vi "OP600ZP_BOITE_DIALOGUE.vi"(0 "Enable":bool=TRUE caption="Activer", 5 "error in (no error)":errorcluster caption="entrée d'erreur (pas d'erreur)") -> (11 "Factory Temperature":dbl format="%#g", 12 "Min Cell Temperature":dbl format="%#g", 13 "Max Cell Temperature":dbl format="%#g", 14 "Min Cell Voltage":dbl format="%#g", 15 "Max Cell Voltage":dbl format="%#g", 16 "Battery Voltage":dbl format="%#g", 17 "PARK Mode OK?":bool, 18 "OK":bool, 19 "error out":errorcluster caption="sortie d'erreur")   [LabVIEW 2020]
doc: "Affiche une boîte de dialogue standard qui invite l'utilisateur à entrer des informations, telles qu'un nom d'utilisateur et un mot de passe.\n--------------------\n\nCe VI Express est configuré comme suit :\n\nMessage à afficher à l'utilisateur :Saisir les valeur suivantes :\nLes entrées sont : \nCase à cocher : PARK Mode OK?\nNombre : Battery Voltage\nNombre : Max Cell Voltage\nNombre : Min Cell Voltage\nNombre : Max Cell Temperature\nNombre : Min Cell Temperature\nNombre : Factory Temperature"
panel:
  out "SOH":dbl caption="Factory Temperature" format="%#g"
  out "SOC":dbl caption="Factory Temperature" format="%#g"
  in  "SOH":dbl caption="Factory Temperature" format="%#g"
  in  "SOC":dbl caption="Factory Temperature" format="%#g"
  in  "Factory Temperature":dbl format="%#g"
  in  "Min Cell Temperature":dbl format="%#g"
  in  "Max Cell Temperature":dbl format="%#g"
  in  "Min Cell Voltage":dbl format="%#g"
  in  "Max Cell Voltage":dbl format="%#g"
  in  "Battery Voltage":dbl format="%#g"
  in  "PARK Mode OK?":bool
  out "String":string="Saisir les valeur suivantes :" caption="Chaîne"
  in  "Cancel":bool caption="Annuler"
  in  "OK2":bool
  in  "OK1":bool
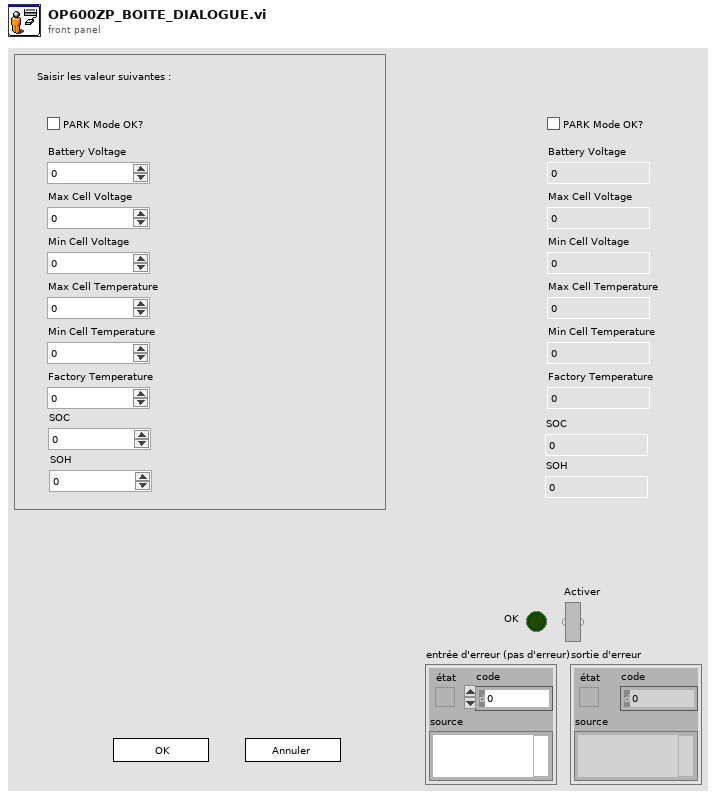
[diagram p1: front panel]
types:
  T1 = cluster{"Input Name":string, "Input Data Type":i32}[]
  T2 = enum8{"Enabled", "Disabled", "Disabled and Grayed Out"}
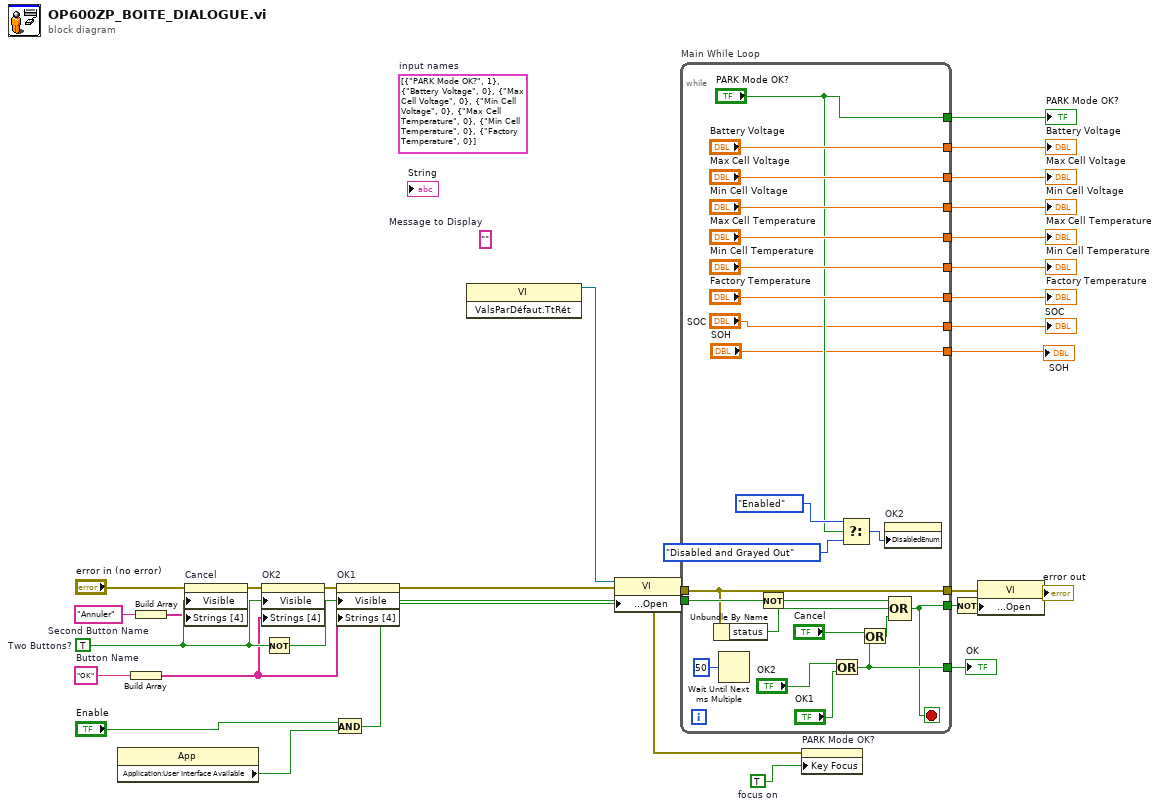
[diagram p0: block diagram]
diagram:
  w11 = TRUE  # focus on
  (unwired) T1 [{"Input Name"="PARK Mode OK?", "Input Data Type"=1}, {"Input Name"="Battery Voltage", "Input Data Type"=0}, {"Input Name"="Max Cell Voltage", "Input Data Type"=0}, {"Input Name"="Min Cell Voltage", "Input Data Type"=0}, {"Input Name"="Max Cell Temperature", "Input Data Type"=0}, {"Input Name"="Min Cell Temperature", "Input Data Type"=0}, {"Input Name"="Factory Temperature", "Input Data Type"=0}]  # input names
  w22 = "Annuler"  # Second Button Name
  w20 = "OK"  # Button Name
  (unwired) ""  # Message to Display
  w30 = TRUE  # Two Buttons?
  n1 = property class="App"() -> ("Application:User Interface Available"=w13:bool)  [unwired: 2 in, 2 out]
  n2 = Build Array(w20) -> (w21:string[])
  n3 = Build Array(w22) -> (w23:string[])
  n4 = property on="Cancel" class="Bool"(error in="error in (no error)", "Visible"=w30, "Strings [4]"=w23) -> (error out=w27:errorcluster)  [unwired: 1 in, 1 out]
  n5 = property on="OK2" class="Bool"(error in=w27, "Visible"=w30, "Strings [4]"=w21) -> (error out=w26:errorcluster)  [unwired: 1 in, 1 out]
  n6 = Not(x=w30) -> (.not. x?=w28:bool)
  n7 = And(x="Enable", y=w13) -> (x .and. y?=w14:bool)
  n8 = property on="OK1" class="Bool"(error in=w26, "Visible"=w28, "Strings [4]"=w21) -> (error out=w3:errorcluster)  [unwired: 1 in, 1 out]
  n9 = invoke class="VI" method="ValsParDéfaut.TtRét"() -> (reference out=w12:refnum<vi>)  [unwired: 3 in, 2 out]
  n10 = property class="VI"(reference=w12, error in=w3, "Front Panel Window:Open"=w14) -> (error out=w19:errorcluster)  [unwired: 1 out]
  n11 = while "Main While Loop" {
    tunnel: [w51] -> w29
    tunnel: w14 -> [w49]
    tunnel: [w47] -> w24
    tunnel: w19 -> [w46]
    tunnel: [w46] -> w17
    tunnel: ["PARK Mode OK?"] -> w4
    tunnel: ["Battery Voltage"] -> w10
    tunnel: ["Max Cell Voltage"] -> w9
    tunnel: ["Min Cell Voltage"] -> w8
    tunnel: ["Max Cell Temperature"] -> w7
    tunnel: ["Min Cell Temperature"] -> w6
    tunnel: ["Factory Temperature"] -> w5
    tunnel: ["SOC"] -> w2
    tunnel: ["SOH"] -> w1
    stop <- w47 stop-if-true
    n12 = Unbundle By Name(w46) -> ("status"=w44:bool)
    n13 = Wait Until Next ms Multiple(millisecond multiple=u32 50) -> ()  [unwired: 1 out]
    n14 = Not(x=w49) -> (.not. x?=w48:bool)
    n15 = Or(x="OK2", y="OK1") -> (x .or. y?=w51:bool)
    n16 = Select(t=T2."Enabled" ("Désactivé"), s="PARK Mode OK?", f=T2."Disabled and Grayed Out" ("Désactivé")) -> (s? t:f=w33:T2)
    n17 = Or(x="Cancel", y=w51) -> (x .or. y?=w45:bool)
    n18 = property on="OK2" class="Bool"("DisabledEnum"=w33) -> ()  [unwired: 2 in, 2 out]
    n19 = Compound Arithmetic op=OR(w48, w44, w45) -> (w47:bool)
  }
  "OK" <- w29
  "PARK Mode OK?" <- w4
  "Battery Voltage" <- w10
  "Max Cell Voltage" <- w9
  "Min Cell Voltage" <- w8
  "Max Cell Temperature" <- w7
  "Min Cell Temperature" <- w6
  "Factory Temperature" <- w5
  "SOC" <- w2
  "SOH" <- w1
  n20 = property on="PARK Mode OK?" class="Bool (strict)"(error in=w19, "Key Focus"=w11) -> ()  [unwired: 1 in, 2 out]
  n21 = Not(x=w24) -> (.not. x?=w25:bool)
  n22 = property class="VI"(error in=w17, "Front Panel Window:Open"=w25) -> (error out=→"error out":errorcluster)  [unwired: 1 in, 1 out]
